vi "Create Test Executive.vi"(8 "error in (no error)":errorcluster, 10 "Create Test Executive":T1, 11 "Test Executive Builder in":refnum<class "Test Executive Builder.lvclass">) -> (0 "error out":errorcluster, 3 "Test Executive Builder out":refnum<class "Test Executive Builder.lvclass">, 5 "Unique ID":string)   [LabVIEW 2019, in "Test Executive Builder.lvclass"]
uses:
  <vilib>/gpm_packages/@cs/Test-executive-builder/Example/Application/Test Executive Builder/Test Executive Builder/Test Executive Builder.lvclass
  C:/Program Files/National Instruments/LabVIEW 2019/vi.lib/gpm_packages/@cs/Test-executive-builder/Source/Test Executive Builder Model/Test Executive Builder Model/Test Executive Builder Model.lvclass
  <vilib>/gpm_packages/@cs/Test-executive-builder/Source/Application Dependencies/Create Test Executive.ctl
  <vilib>/gpm_packages/@cs/Test-executive-builder/Source/Test Executive Builder Model/Test Executive Builder Model/Test Executive Builder Model.lvclass/Test Executive Builder Model.ctl
  <vilib>/gpm_packages/@cs/Test-executive-builder/Example/Application/Test Executive Builder/Test Executive Builder/Test Executive Builder.lvclass/Test Executive Builder.ctl
  cf7b5331-a396-4611-81c8-c822f2fb9f9c.vi
  <vilib>/Utility/error.llb/Error Cluster From Error Code.vi
  <vilib>/gpm_packages/@cs/Test-executive-builder/Source/Test Executive Builder Model/Test Executive Builder Model/Test Executive Builder Model.lvclass
  <vilib>/gpm_packages/@cs/test-executive/Source/Test Executive/ITestExecutive/ITest Executive.lvclass
  <vilib>/gpm_packages/@cs/Test-executive-builder/Source/Test Executive Builder Dialogs/ITest Executive Builder Dialog/ITest Executive Builder Dialog.lvclass
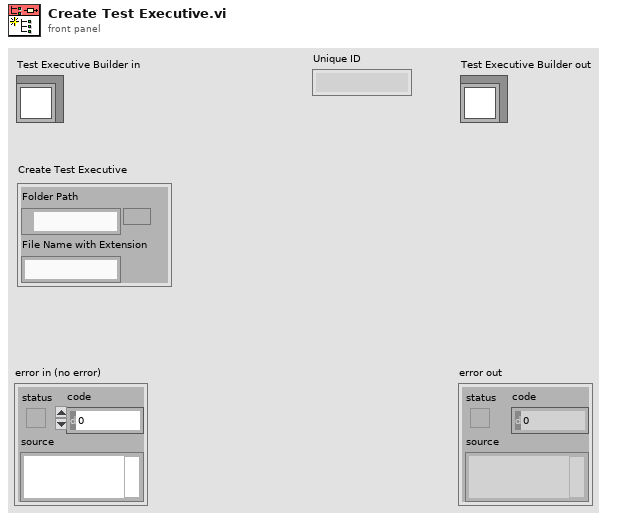
[diagram p1: front panel]
types:
  T1 = typedef "Create Test Executive.ctl" = cluster{"Folder Path":path, "File Name with Extension":string}
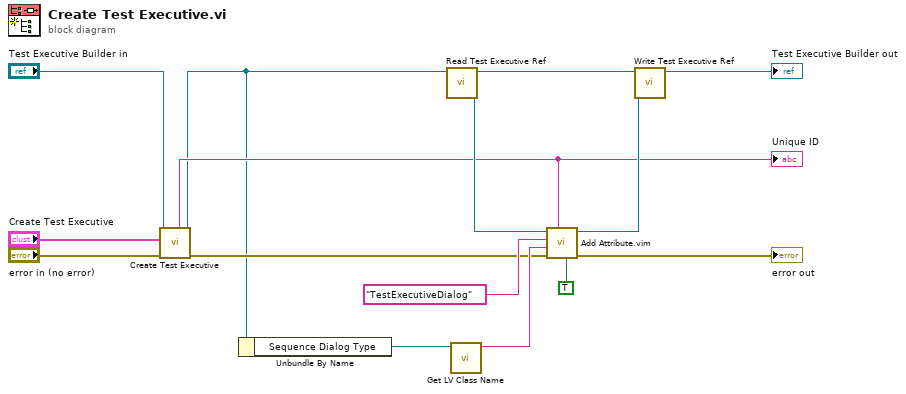
[diagram p0: block diagram]
diagram:
  n1 = call-parent "Create Test Executive.vi"("error in (no error)"="error in (no error)", "Create Test Executive"="Create Test Executive", "Test Executive Builder Model in"="Test Executive Builder in") -> ("error out"=w6:errorcluster, "Test Executive Builder Model out"=w2:refnum<class "Test Executive Builder.lvclass">, "Unique ID"=w5:string)  [unwired: 6 in]
  "Unique ID" <- w5
  n2 = Unbundle By Name(w2) -> ("Sequence Dialog Type"=w1:refnum<class "ITest Executive Builder Dialog.lvclass">)
  n3 = call <vilib>:"Read Test Executive Ref.vi"("Test Executive Builder Model in"=w2) -> ("Test Executive Ref"=w11:refnum<data-value>, "Test Executive Builder Model out"=w12:refnum<class "Test Executive Builder.lvclass">)  [unwired: 9 in]
  n4 = call <vilib>:"Get LV Class Name.vi"("object"=w1) -> ("class name"=w7:string)  [unwired: 9 in, 1 out]
  n5 = call "Add Attribute.vim"("Private?"=TRUE, "ID"=w5, "error in (no error)"=w6, "Attribute"=w7, "Attribute Name"="TestExecutiveDialog", "Test Executive Ref"=w11) -> ("error out"=→"error out":errorcluster, "Test Executive Ref out"=w10:refnum<data-value>)  [unwired: 2 in, 2 out]
  n6 = call <vilib>:"Write Test Executive Ref.vi"("Test Executive Ref"=w10, "Test Executive Builder Model in"=w12) -> ("Test Executive Builder Model out"=→"Test Executive Builder out":refnum<class "Test Executive Builder.lvclass">)  [unwired: 9 in]
